vi "1.3-What.vi"   [LabVIEW 2010]
uses:
  2-Low Neurons/2.3-What Sensor Typedef.ctl
  2-Low Neurons/Data Latch.ctl
  1.0-Hindbrain Global.vi
types:
  T1 = typedef "2.3-What Sensor Typedef.ctl" = cluster{"FPGA Raw Datalatch":T2, "Drivable Path Integers":u16[]}
  T2 = typedef "Data Latch.ctl" = enum8{"Idle", "Sending", "Sent", "Receiving", "Received"}
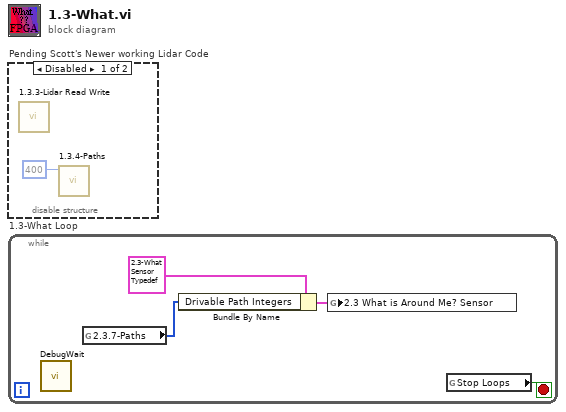
[diagram p0: block diagram]
diagram:
  n1 = disable-structure "Pending Scott's Newer working Lidar Code" shown="Disabled" {
    frame Disabled {
      n2 = call "1.3.3-Lidar Read Write.vi"() -> ()  [unwired: 1 in]
      n3 = call "1.3.4-Paths.vi"("allowed proximity squared"=i16 400) -> ()  [unwired: 11 in]
    }
    frame Enabled {
    }
  }
  n4 = while "1.3-What Loop" {
    stop <- w5 stop-if-true
    n5 = call "DebugWait.vi"() -> ()  [unwired: 12 in]
    n6 = global read "1.0-Hindbrain Global.vi" "2.3.7-Paths"() -> (w3:u16[])
    n7 = Bundle By Name(cluster=T1 {"FPGA Raw Datalatch"=enum."Idle", "Drivable Path Integers"=[0, 0, 0, 0, 0, 0, 0, 0, 0, 0, 0, 0, 0, 0, 0, 0]} ("2.3 What is Around Me? Sensor"), "Drivable Path Integers"=w3) -> (w2:T1)
    n8 = global write "1.0-Hindbrain Global.vi" "2.3 What is Around Me? Sensor"(w2) -> ()
    n9 = global read "1.0-Hindbrain Global.vi" "Stop Loops"() -> (w5:bool)
  }
